vi "updateSums.vi"(8 "error in (no error)":errorcluster, 9 "col":u8, 10 "row":u8, 11 "BingoBoard in":refnum<class "BingoBoard.lvclass">) -> (0 "error out":errorcluster, 2 "won?":bool, 3 "BingoBoard out":refnum<class "BingoBoard.lvclass">)   [LabVIEW 2017, in "BingoBoard.lvclass"]
uses:
  BingoBoard.lvclass
  BingoBoard.lvclass/BingoBoard.ctl
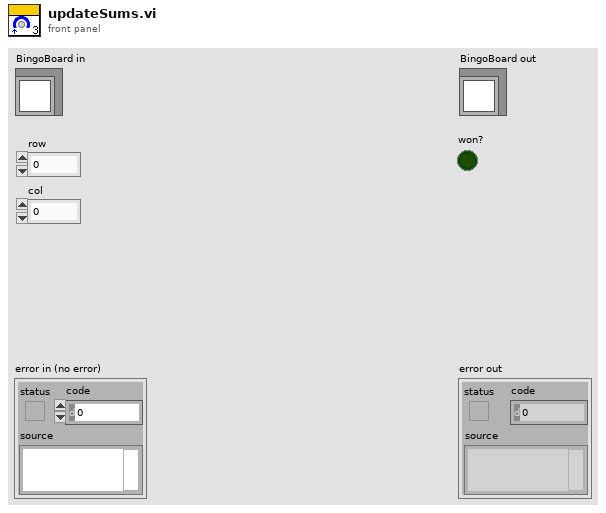
[diagram p1: front panel]
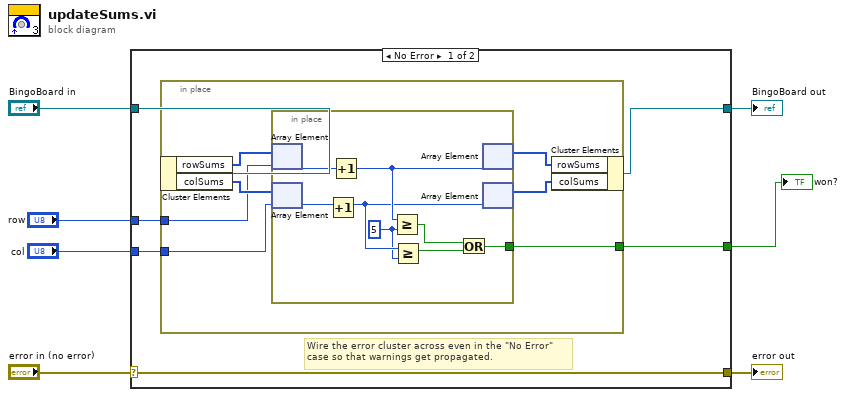
[diagram p0: block diagram]
diagram:
  n1 = case shown="No Error" "error in (no error)" {
    selector: "error in (no error)" -> [w13 w30]
    tunnel: [w13 w30] -> w6
    tunnel: [w11 w29] -> w4
    tunnel: "BingoBoard in" -> [w12 w29]
    tunnel: "row" -> [w10 _]
    tunnel: "col" -> [w9 _]
    tunnel: [w8 _] -> w1
    frame No Error {
      # "Wire the error cluster across even in the \"No Error\"\ncase so that warnings get propagated."
      n2 = in-place {
        in-place-border: w10 -> [w18]
        in-place-border: w9 -> [w17]
        in-place-border: [w16] -> w8
        n3 = in-place-cluster #1(w12) -> ("rowSums"=w20:i32[], "colSums"=w19:i32[])
        n4 = in-place {
          in-place-border: [w21] -> w16
          w24 = 5 ("y")
          n5 = in-place-array #2(w20, w18) -> (w28:i32)
          n6 = in-place-array #3(w19, w17) -> (w27:i32)
          n7 = Increment(x=w27) -> (x+1=w25:i32)
          n8 = Increment(x=w28) -> (x+1=w26:i32)
          n9 = Greater Or Equal?(x=w26, y=w24) -> (x >= y?=w23:bool)
          n10 = Greater Or Equal?(x=w25, y=w24) -> (x >= y?=w22:bool)
          n11 = Or(x=w23, y=w22) -> (x .or. y?=w21:bool)
          n12 = in-place-array #2(w26) -> (w15:i32[])  [unwired: 1 out]
          n13 = in-place-array #3(w25) -> (w14:i32[])  [unwired: 1 out]
        }
        n14 = in-place-cluster #1("rowSums"=w15, "colSums"=w14) -> (w11:refnum<class "BingoBoard.lvclass">)
      }
    }
    frame Error {
    }
  }
  "error out" <- w6
  "BingoBoard out" <- w4
  "won?" <- w1
